vi "Get Log Item by ID.vi"(8 "error in (no error)":errorcluster, 10 "ID":u32, 11 "Debug Log In":refnum<class "Debug Log.lvclass">) -> (0 "error out":errorcluster, 2 "Data Log":refnum<class "Debug Data.lvclass">, 3 "Debug Log Out":refnum<class "Debug Log.lvclass">)   [LabVIEW 2020, in "Debug Log.lvclass"]
uses:
  Debug Log.lvclass
  Debug Data/Debug Data.lvclass
  Debug Log.lvclass/Debug Log.ctl
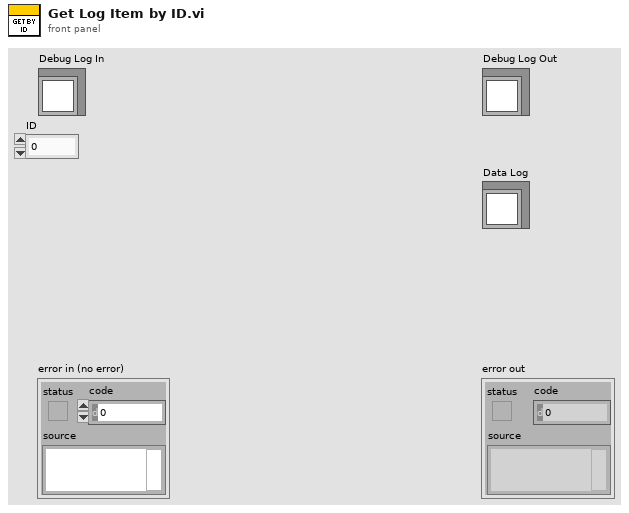
[diagram p1: front panel]
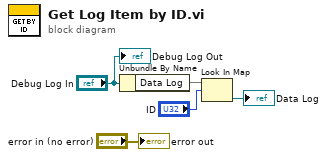
[diagram p0: block diagram]
diagram:
  n1 = Unbundle By Name("Debug Log In") -> ("Data Log"=w3:map{u32, refnum<class "Debug Data.lvclass">})
  n2 = Look In Map(map=w3, key="ID") -> (value=→"Data Log":refnum<class "Debug Data.lvclass">)  [unwired: 1 in, 1 out]
  "error out" <- "error in (no error)"
  "Debug Log Out" <- "Debug Log In"
